vi "DigitToStr.vi"(11 "时/分":u16) -> (3 "00字符串":string)   [LabVIEW 2014]
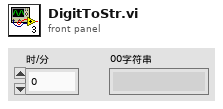
[diagram p1: front panel]
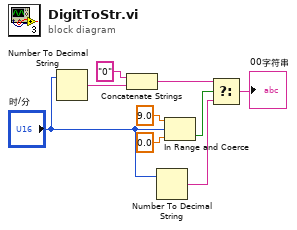
[diagram p0: block diagram]
diagram:
  n1 = Number To Decimal String(number="时/分") -> (decimal integer string=w6:string)  [unwired: 1 in]
  n2 = Concatenate Strings("0", w6) -> (w8:string)
  n3 = Number To Decimal String(number="时/分") -> (decimal integer string=w5:string)  [unwired: 1 in]
  n4 = In Range and Coerce(upper limit=9.0 ("上限"), x="时/分", lower limit=0.0 ("下限")) -> (In Range?=w3:bool)  [unwired: 1 out]
  n5 = Select(t=w8, s=w3, f=w5) -> (s? t:f=→"00字符串":string)
